vi "ep_Speed Estimation Check Data Vaild.vi"(0 "waveforms":waveform(dbl)[](array[waveform]), 2 "reset? (F)":bool, 5 "fundamental frequency [Hz]":dbl, 7 "speed estimation settings":cluster{"% overlap":dbl, "algorithm":T1}={"% overlap"=0.0, "algorithm"=enum."3-phase signals"}, 9 "nameplate information":T2, 11 "error in (no error)":errorcluster, 12 "window length [s]":dbl) -> (3 "number of speed":i32, 4 "signals":dbl[][](array[numeric]), 6 "spectra parameters":T3, 8 "dup speed estimation settings":cluster{"% overlap":dbl, "algorithm":T1}={"% overlap"=0.0, "algorithm"=enum."3-phase signals"}, 15 "error out":errorcluster)   [LabVIEW 2014, in "NI_EP_Motor Monitoring.lvlib"]
uses:
  <vilib>/addons/Electrical Power/Motor Monitoring/NI_EP_Motor Monitoring.lvlib
  <vilib>/addons/Electrical Power/Motor Monitoring/subVIs/ep_Demodulation Algorithm.ctl
  <vilib>/addons/Electrical Power/Power Measurement/NI_EP_Power Measurement.lvlib
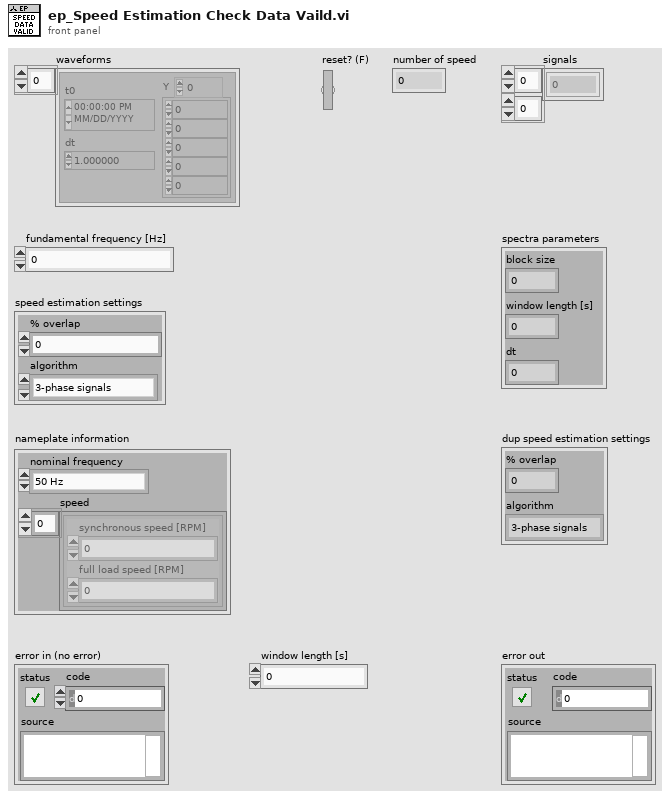
[diagram p1: front panel]
types:
  T1 = typedef "NI_EP_Motor Monitoring.lvlib/ep_Demodulation Algorithm.ctl" = enum16{"1-phase signal", "3-phase signals"}
  T2 = cluster{"nominal frequency":enum16{"50 Hz", "60 Hz"}, "speed":cluster{"synchronous speed [RPM]":dbl, "full load speed [RPM]":dbl}[]}
  T3 = cluster{"block size":i32, "window length [s]":dbl, "dt":dbl}
  T4 = cluster{"synchronous speed [RPM]":dbl, "full load speed [RPM]":dbl}[]
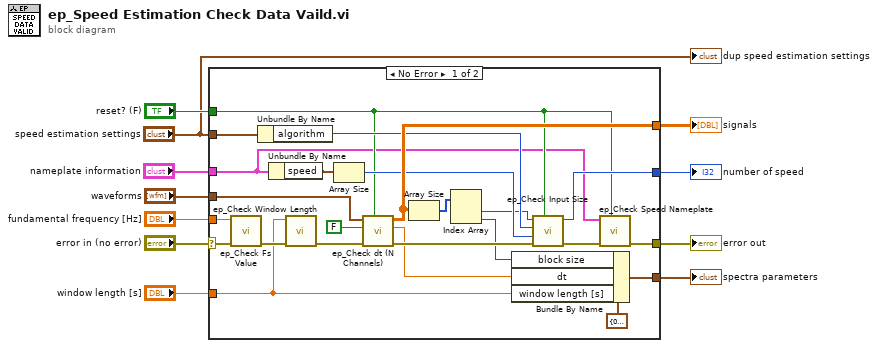
[diagram p0: block diagram]
diagram:
  n1 = case shown="No Error" "error in (no error)" {
    selector: "error in (no error)" -> [w26 w36]
    tunnel: "waveforms" -> [w34 _]
    tunnel: "reset? (F)" -> [w23 _]
    tunnel: "nameplate information" -> [w20 _]
    tunnel: "speed estimation settings" -> [w17 _]
    tunnel: [w32 _] -> w8
    tunnel: "window length [s]" -> [w12 _]
    tunnel: [w29 w36] -> w6
    tunnel: [w25 _] -> w5
    tunnel: "fundamental frequency [Hz]" -> [w24 _]
    tunnel: [w21 _] -> w3
    frame No Error {
      n2 = call <vilib>:"ep_Check Fs Value.vi"("error in (no error)"=w26, "fundamental frequency [Hz]"=w24) -> ("error out"=w14:errorcluster)  [unwired: 9 in]
      n3 = Unbundle By Name(w17) -> ("algorithm"=w28:T1)
      n4 = Unbundle By Name(w20) -> ("speed"=w19:T4)
      n5 = call <vilib>:"ep_Check Window Length.vi"("error in (no error)"=w14, "window length [s]"=w12) -> ("error out"=w13:errorcluster)  [unwired: 9 in]
      n6 = Array Size(array=w19) -> (size(s)=w31:i32)
      n7 = call <vilib>:"ep_Check dt (N Channels).vi"("reset? (F)"=w23, "error in (no error)"=w13, "waveforms only? (F)"=FALSE, "waveforms"=w34) -> ("error out"=w18:errorcluster, "dt"=w15:dbl, "signals"=w32:dbl[][])  [unwired: 3 in, 2 out]
      n8 = Array Size(array=w32) -> (size(s)=w33:i32[])
      n9 = Index Array(array=w33) -> (element #1=w27:i32, element #2=w16:i32)  [unwired: 2 in]
      n10 = Bundle By Name(cluster=T3 {"block size"=0, "window length [s]"=0.0, "dt"=0.0}, "block size"=w16, "dt"=w15, "window length [s]"=w12) -> (w21:T3)
      n11 = call <vilib>:"ep_Check Input Size.vi"("check? (F)"=w23, "error in (no error)"=w18, "array size of nameplate data"=w31, "algorithm"=w28, "number of channels"=w27) -> ("error out"=w30:errorcluster, "number of speed"=w25:i32)  [unwired: 5 in]
      n12 = call <vilib>:"ep_Check Speed Nameplate.vi"("check? (F)"=w23, "error in (no error)"=w30, "nameplate information"=w20) -> ("error out"=w29:errorcluster)  [unwired: 8 in]
    }
    frame Error {
    }
  }
  "error out" <- w6
  "signals" <- w8
  "number of speed" <- w5
  "spectra parameters" <- w3
  "dup speed estimation settings" <- "speed estimation settings"
